vi "beginTableWithStrikerPlay.vi"(10 "Game":refnum<class "Game.lvclass">, 11 "TableWithStrikerPlay in":refnum<class "TableWithStrikerPlay.lvclass">) -> (2 "BeginTableWithStriker?":bool, 3 "TableWithStrikerPlay out":refnum<class "TableWithStrikerPlay.lvclass">)   [LabVIEW 2023, in "TableWithStrikerPlay.lvclass"]
uses:
  TableWithStrikerPlay.lvclass
  Game_class/Game.lvclass
  Referee_class/command_interpreted.ctl
  Team_class/OffensivePlay.ctl
  Game_class/Game.lvclass/Game.ctl
  Team_class/Team.lvclass/Team.ctl
  Referee_class/Referee.lvclass/Referee.ctl
  Game_class/Read Referee.vi
  Game_class/Read Utilities.lvclass.vi
  Referee_class/Read command_interpreted.vi
  Game_class/Read OffensiveTeam.vi
  Team_class/Read RobotRef.vi
  Team_class/Read OffensivePlay.vi
  Ally_class/Ally.lvclass
  Robot_class/Robot.lvclass
  Referee_class/Referee.lvclass
  Utilities_class/Utilities.lvclass
panel:
  out "error out":errorcluster
  in  "error in (no error)":errorcluster
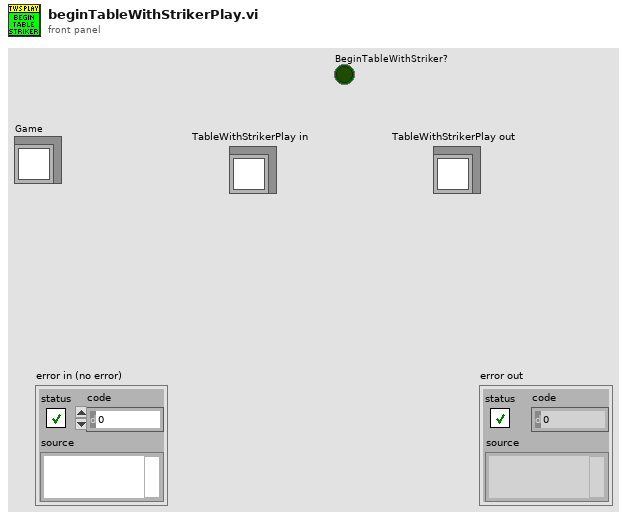
[diagram p1: front panel]
types:
  T1 = typedef "OffensivePlay.ctl" = enum16{"TableWithStriker", "TableWith2ndStrikerPlay", "PrepareDoublePass", "PrepareRollToPass", "SimplePass", "PreparePass", "PassToStriker", "BallOutOfField", "PassTo2ndStriker", "StopOffensive", "Prepare Penalty Enemy", "EnemyPossessionAtEnemyField", "EnemyPossesionAtOurField", "TestPlay", "PreparePenaltyAlly", "KickPenaltyAlly", "PrepareKickoffAlly", "PrepareKickoffEnemy", "IndirectEnemy", "DirectEnemy", "NormalGame", "DirectKick", "Pass", "Halt", "Timeout", "PassPlay", "PenaltyEnemy"}
  T2 = typedef "command_interpreted.ctl" = enum16{"Goal Ally", "Goal Enemy", "Ball Placement Enemy", "Ball Placement Ally", "Normal Half Time", "Extra Time  Break", "Extra Half Time", "None", "Post Game", "PKA Normal Start", "Prepare Kickoff Ally", "PKE Normal Start", "Prepare Kickoff Enemy", "Force Start", "Halt", "Timeout", "Prepare Penalty Ally", "Prepare Penalty Enemy", "PPA NormalStart", "PPE Normal Start", "Indirect Free Ally", "Direct Free Enemy", "Direct Free Ally", "Indirect Free Enemy", "Stop"}
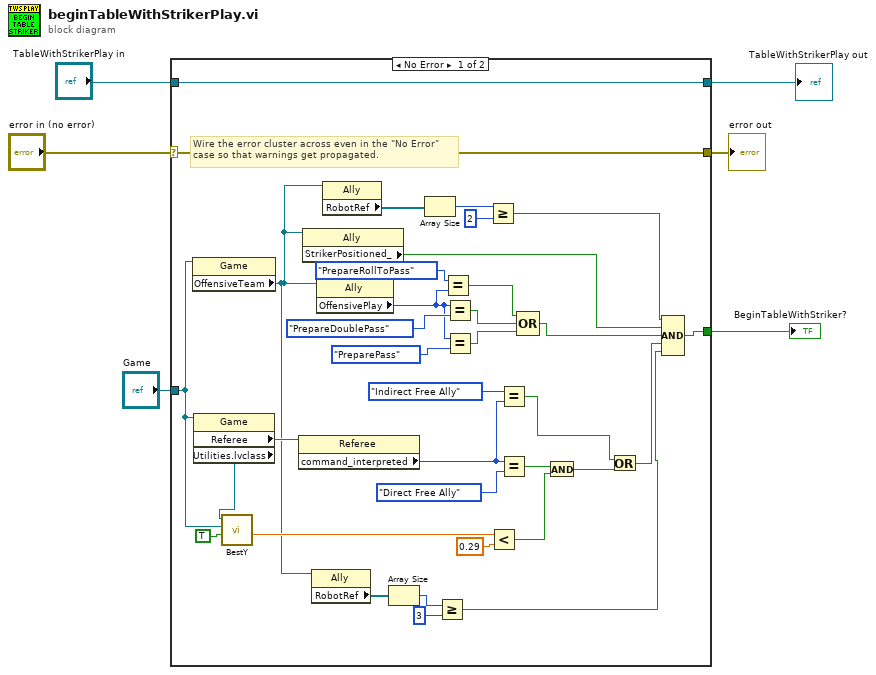
[diagram p0: block diagram]
diagram:
  n1 = case shown="No Error" "error in (no error)" {
    selector: "error in (no error)" -> [w40 w43]
    tunnel: [w40 w43] -> w5
    tunnel: [w41 w42] -> w1
    tunnel: "TableWithStrikerPlay in" -> [w41 w42]
    tunnel: "Game" -> [w31 _]
    tunnel: [w30 _] -> w3
    frame No Error {
      # "Wire the error cluster across even in the \"No Error\"\ncase so that warnings get propagated."
      n2 = property class="Game"(reference=w31) -> ("OffensiveTeam"=w8:refnum<class "Ally.lvclass">)  [unwired: 1 in, 2 out]
      n3 = property class="Game"(reference=w31) -> ("Referee"=w39:refnum<class "Referee.lvclass">, "Utilities.lvclass"=w15:refnum<class "Utilities.lvclass">)  [unwired: 1 in, 2 out]
      n4 = call "BestY.vi"("Utilities in"=w15, "Game"=w31, "inimigos"=TRUE) -> ("Gap kick"=w33:dbl)  [unwired: 2 in, 4 out]
      n5 = property class="Referee"(reference=w39) -> ("command_interpreted"=w37:T2)  [unwired: 1 in, 2 out]
      n6 = property class="Ally"(reference=w8) -> ("StrikerPositioned_"=w29:bool)  [unwired: 1 in, 2 out]
      n7 = property class="Ally"(reference=w8) -> ("RobotRef"=w11:refnum<class "Robot.lvclass">[])  [unwired: 1 in, 2 out]
      n8 = property class="Ally"(reference=w8) -> ("OffensivePlay"=w14:T1)  [unwired: 1 in, 2 out]
      n9 = property class="Ally"(reference=w8) -> ("RobotRef"=w20:refnum<class "Robot.lvclass">[])  [unwired: 1 in, 2 out]
      n10 = Array Size(array=w11) -> (size(s)=w10:i32)
      n11 = Array Size(array=w20) -> (size(s)=w19:i32)
      n12 = Greater Or Equal?(x=w10, y=3) -> (x >= y?=w7:bool)
      n13 = Equal?(x=OffensivePlay."PrepareRollToPass" ("OffensivePlay"), y=w14) -> (x = y?=w22:bool)
      n14 = Equal?(x=w14, y=OffensivePlay."PrepareDoublePass" ("OffensivePlay")) -> (x = y?=w23:bool)
      n15 = Equal?(x=w14, y=OffensivePlay."PreparePass" ("OffensivePlay")) -> (x = y?=w12:bool)
      n16 = Greater Or Equal?(x=w19, y=2) -> (x >= y?=w17:bool)
      n17 = Less?(x=w33, y=0.29 ("Gap kick")) -> (x < y?=w32:bool)
      n18 = Equal?(x=command_interpreted."Indirect Free Ally" ("command_interpreted"), y=w37) -> (x = y?=w26:bool)
      n19 = Equal?(x=w37, y=command_interpreted."Direct Free Ally" ("command_interpreted")) -> (x = y?=w28:bool)
      n20 = Compound Arithmetic op=OR(w22, w23, w12) -> (w21:bool)
      n21 = And(x=w28, y=w32) -> (x .and. y?=w27:bool)
      n22 = Or(x=w26, y=w27) -> (x .or. y?=w16:bool)
      n23 = Compound Arithmetic op=AND(w17, w29, w21, w16, w7) -> (w30:bool)
    }
    frame Error {
    }
  }
  "error out" <- w5
  "BeginTableWithStriker?" <- w3
  "TableWithStrikerPlay out" <- w1
